vi "ProtocolControl_QMH.vi"() -> ()   [LabVIEW 2015]
uses:
  ProtocolStatus.ctl
  <vilib>/xml/Close Reference(Node).vi
  <vilib>/xml/Load XML File.vi
  <vilib>/xml/NI_XML.lvlib
  <resource>/objmgr/DOMUserDefRef.rc
panel:
  out "Current Subsession":string caption="Name"
  out "Time of Current Subsession":dbl caption="Time"
  out "Current Subsession Idx":i32 caption="Index"
  in  "Engage":bool
  in  "Subject ID":string
  out "Time to Next Subsession":dbl
  out "Pause Time":dbl
  out "Record Time":dbl
  out "Session Time (s)":dbl
  out "Current Session":dbl(slide) min=0.0 max=600.0 scale=0.0..180.0
  out "Current Time":dbl
  out "File Name":string
  out "Suggestions":string
  in  "Close Protocol":bool
  in  "Pause Session":bool
  in  "Start Session":bool
  in  "Load Protocol":bool
  in  "Sessions":i32(listbox)
  out "parse errors":string
  in  "XML File Path":path=path "D:/JinXin/LabVIEW.git/CAlex2-Controller/Remote VIs/Protocol/TrainingProtocol.xml"
  # "Subsession"
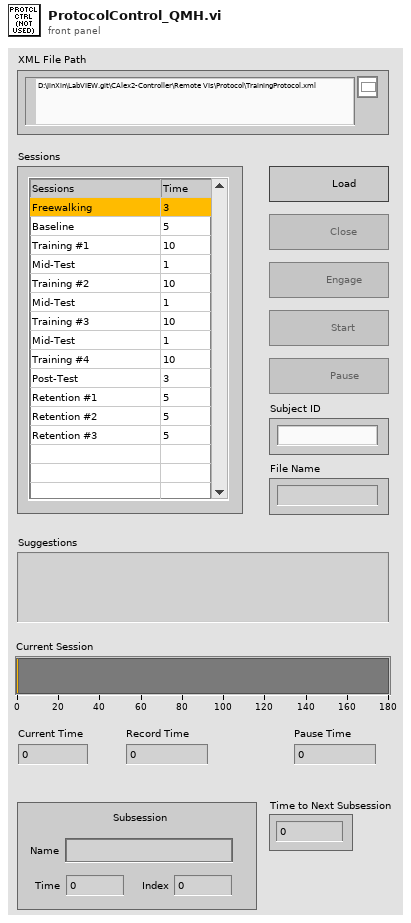
[diagram p1: front panel]
types:
  T1 = typedef "ProtocolStatus.ctl" = enum16{"No Protocol", "Protocol Idle", "Protocol Start", "Protocol Pause"}
  T2 = enum8{"Enabled", "Disabled", "Disabled and Grayed Out"}
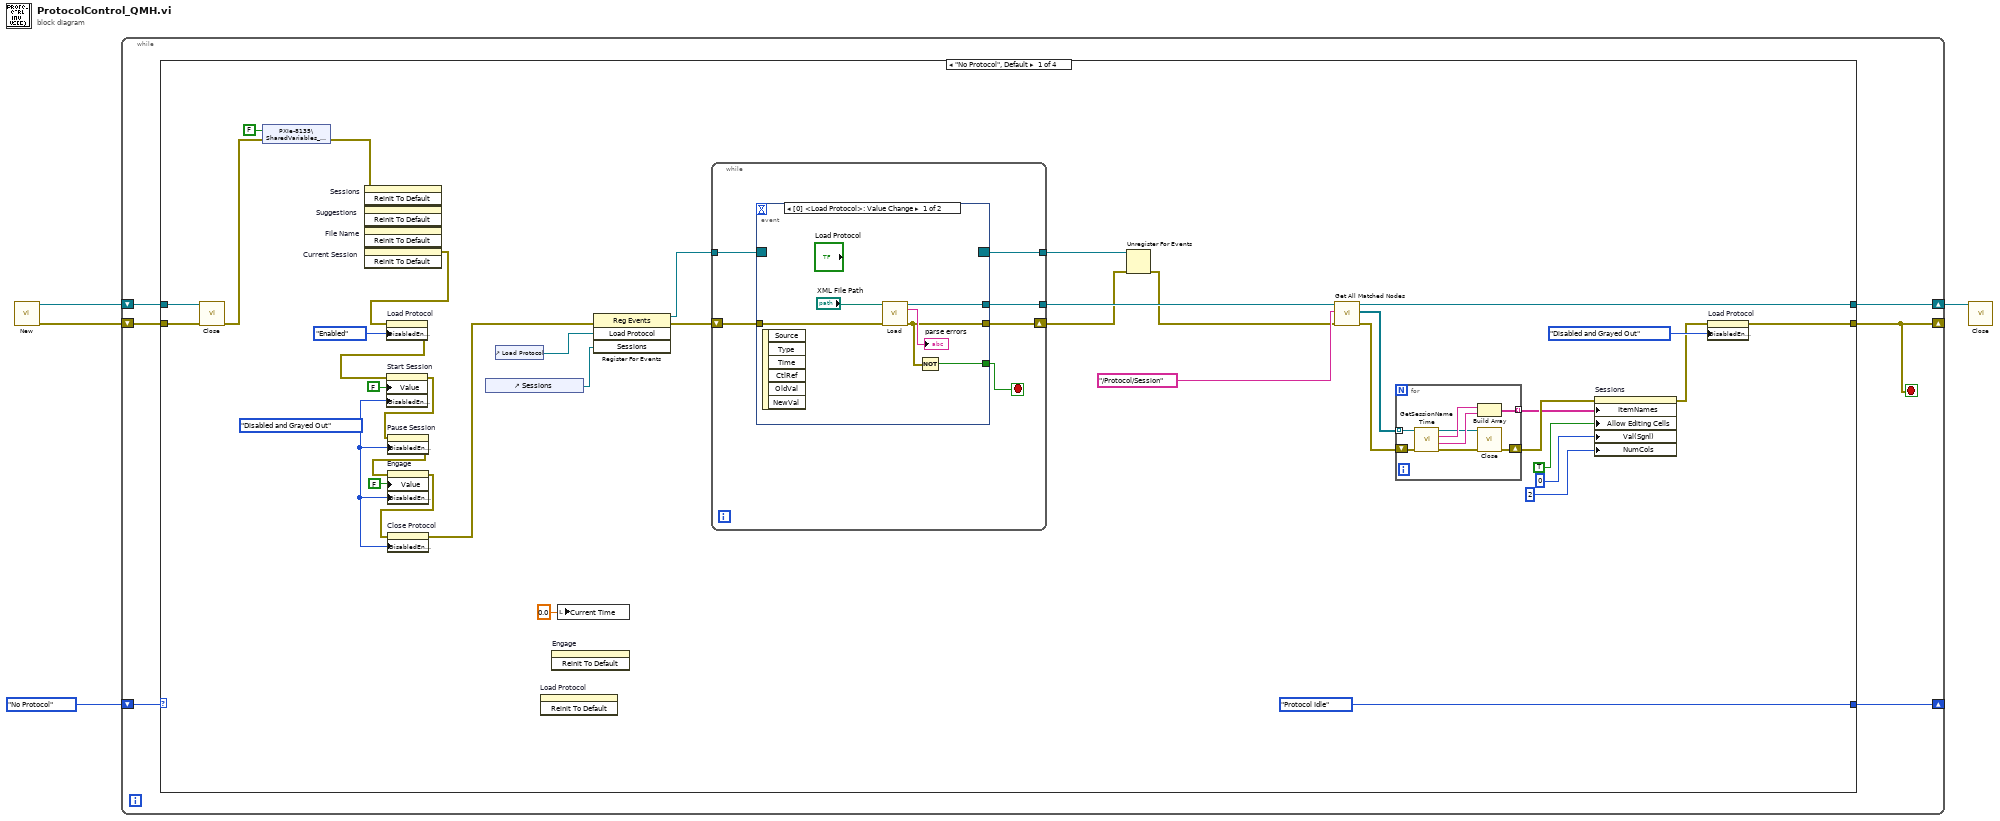
[diagram p0: block diagram]
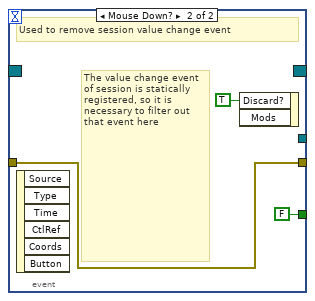
[diagram p2: hidden frame]
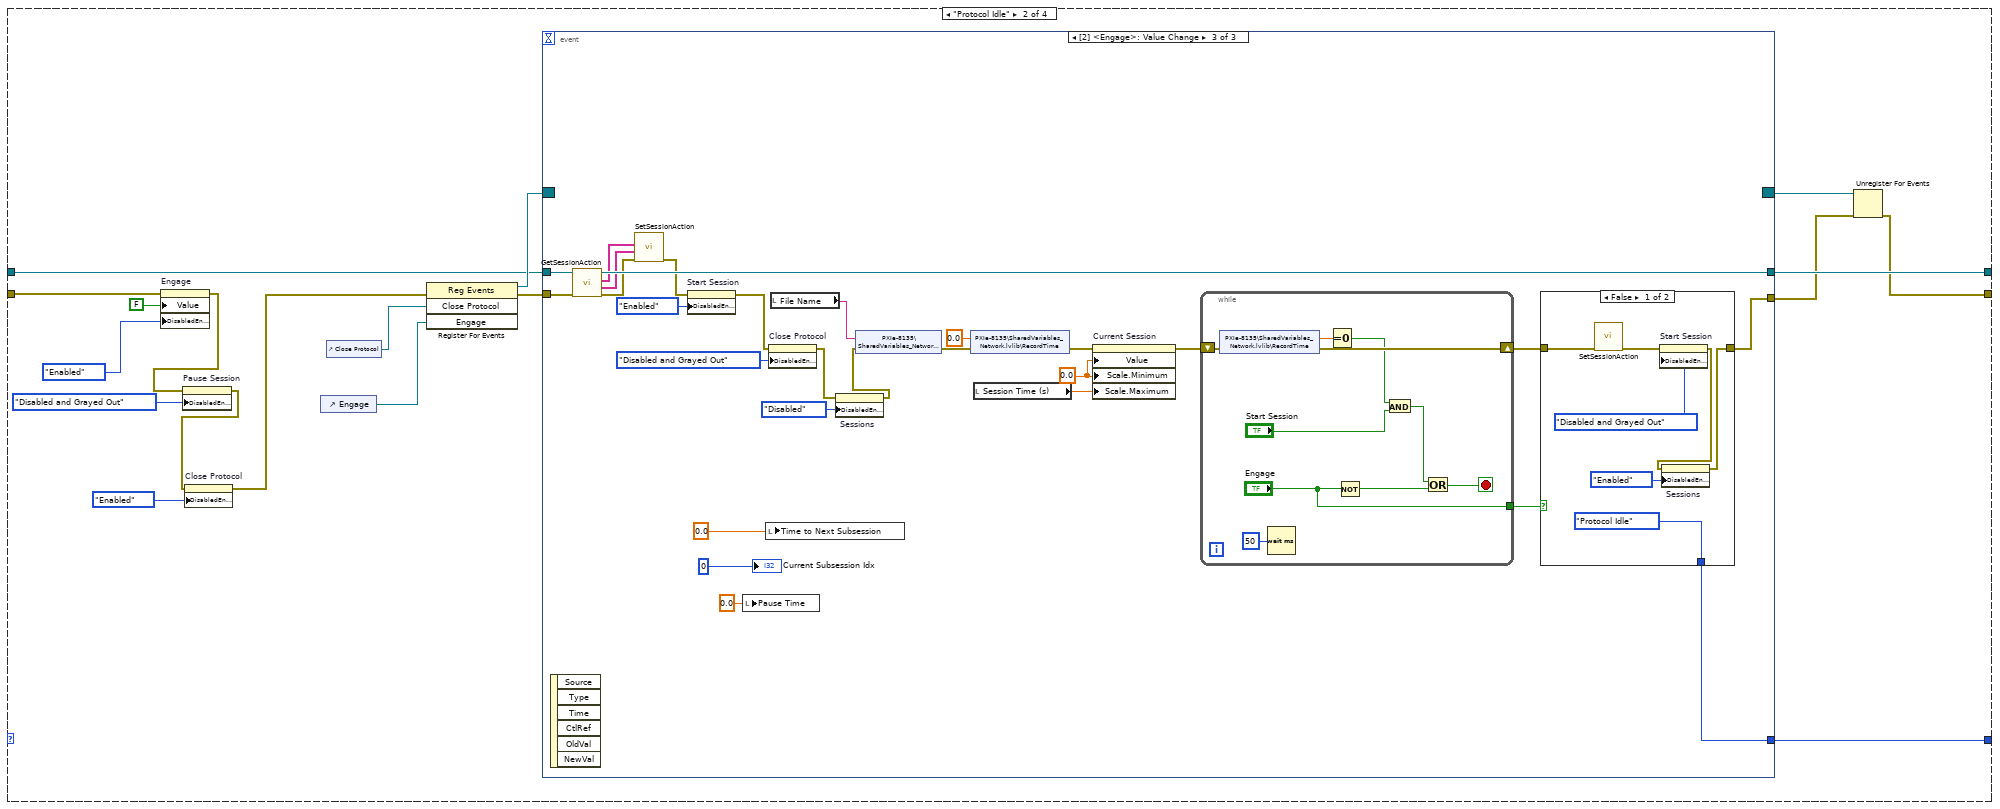
[diagram p3: hidden frame]
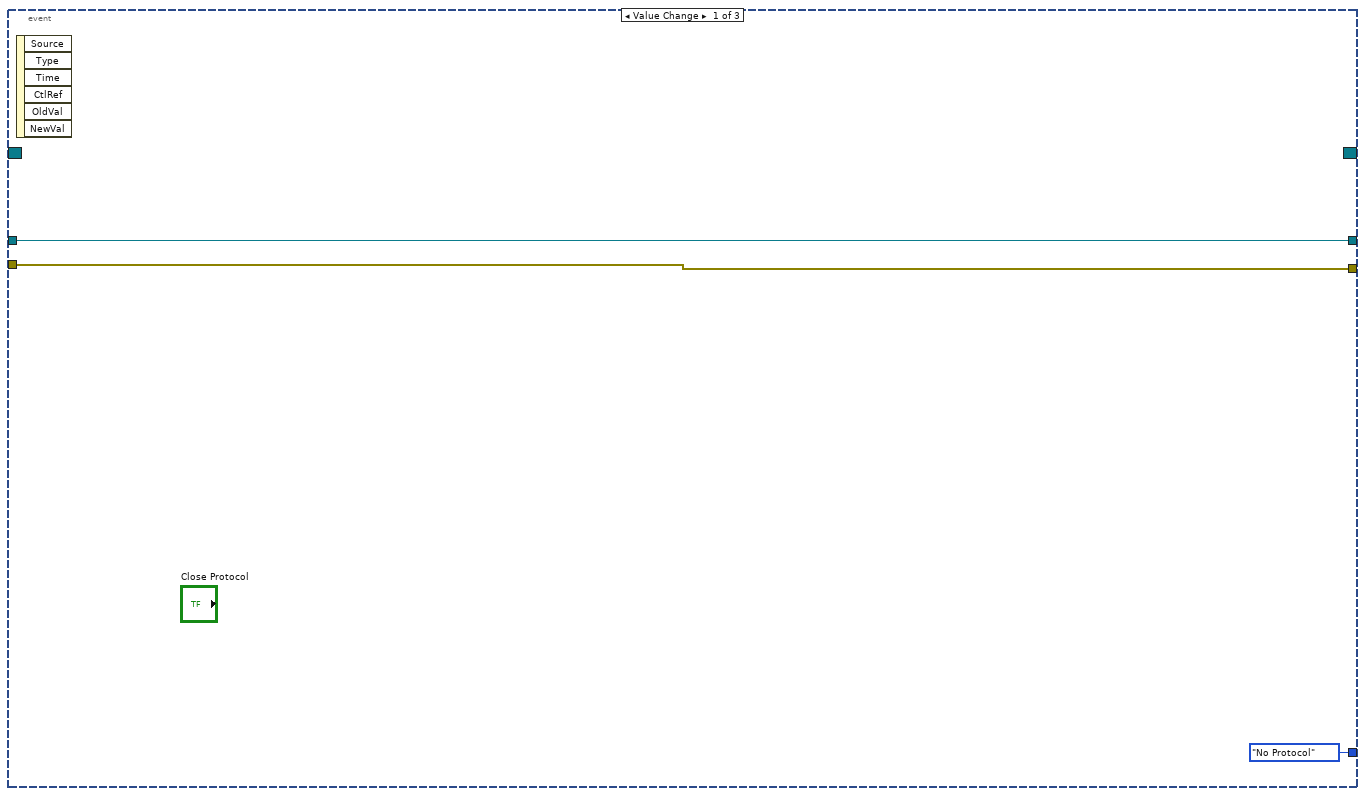
[diagram p4: hidden frame]
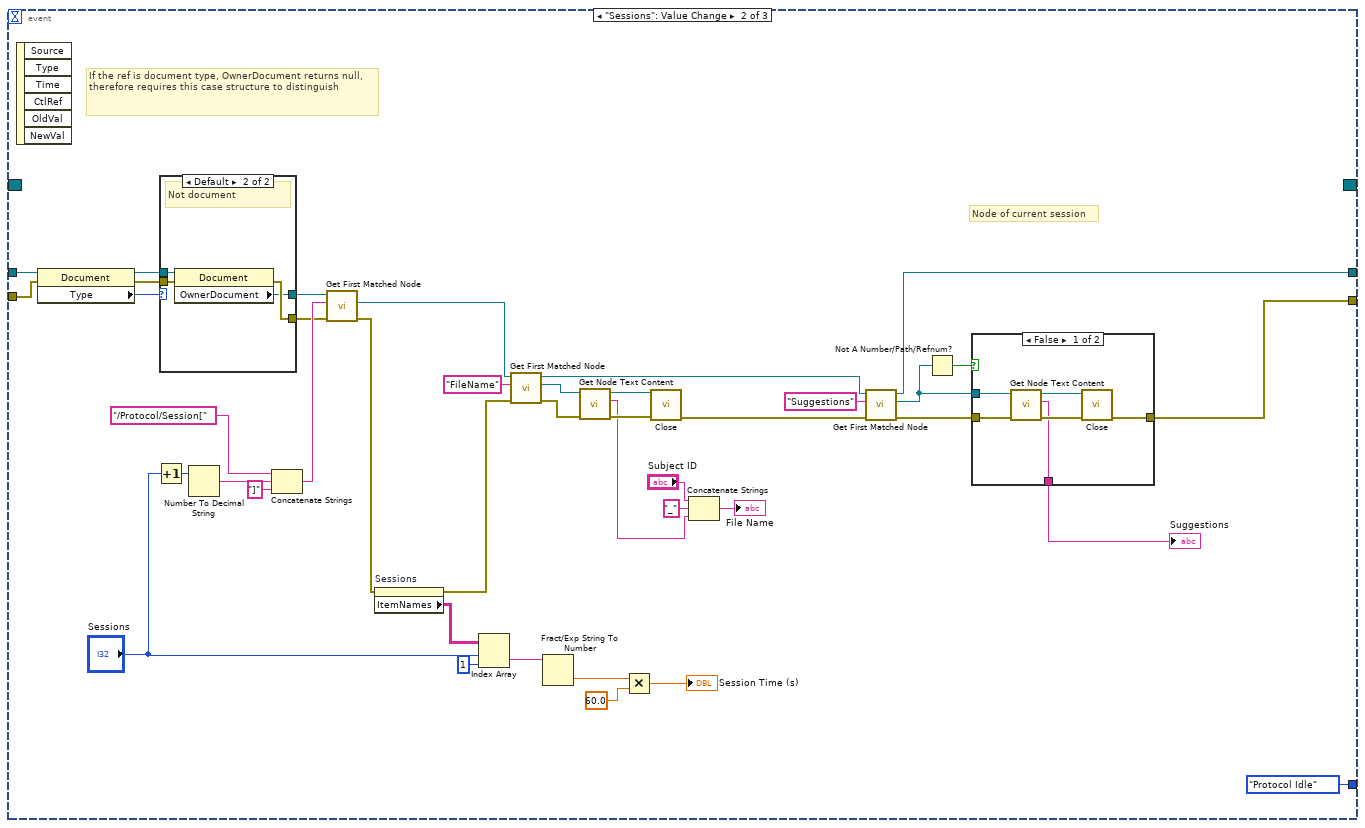
[diagram p5: hidden frame]
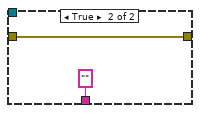
[diagram p7: hidden frame]
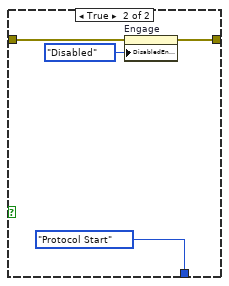
[diagram p8: hidden frame]
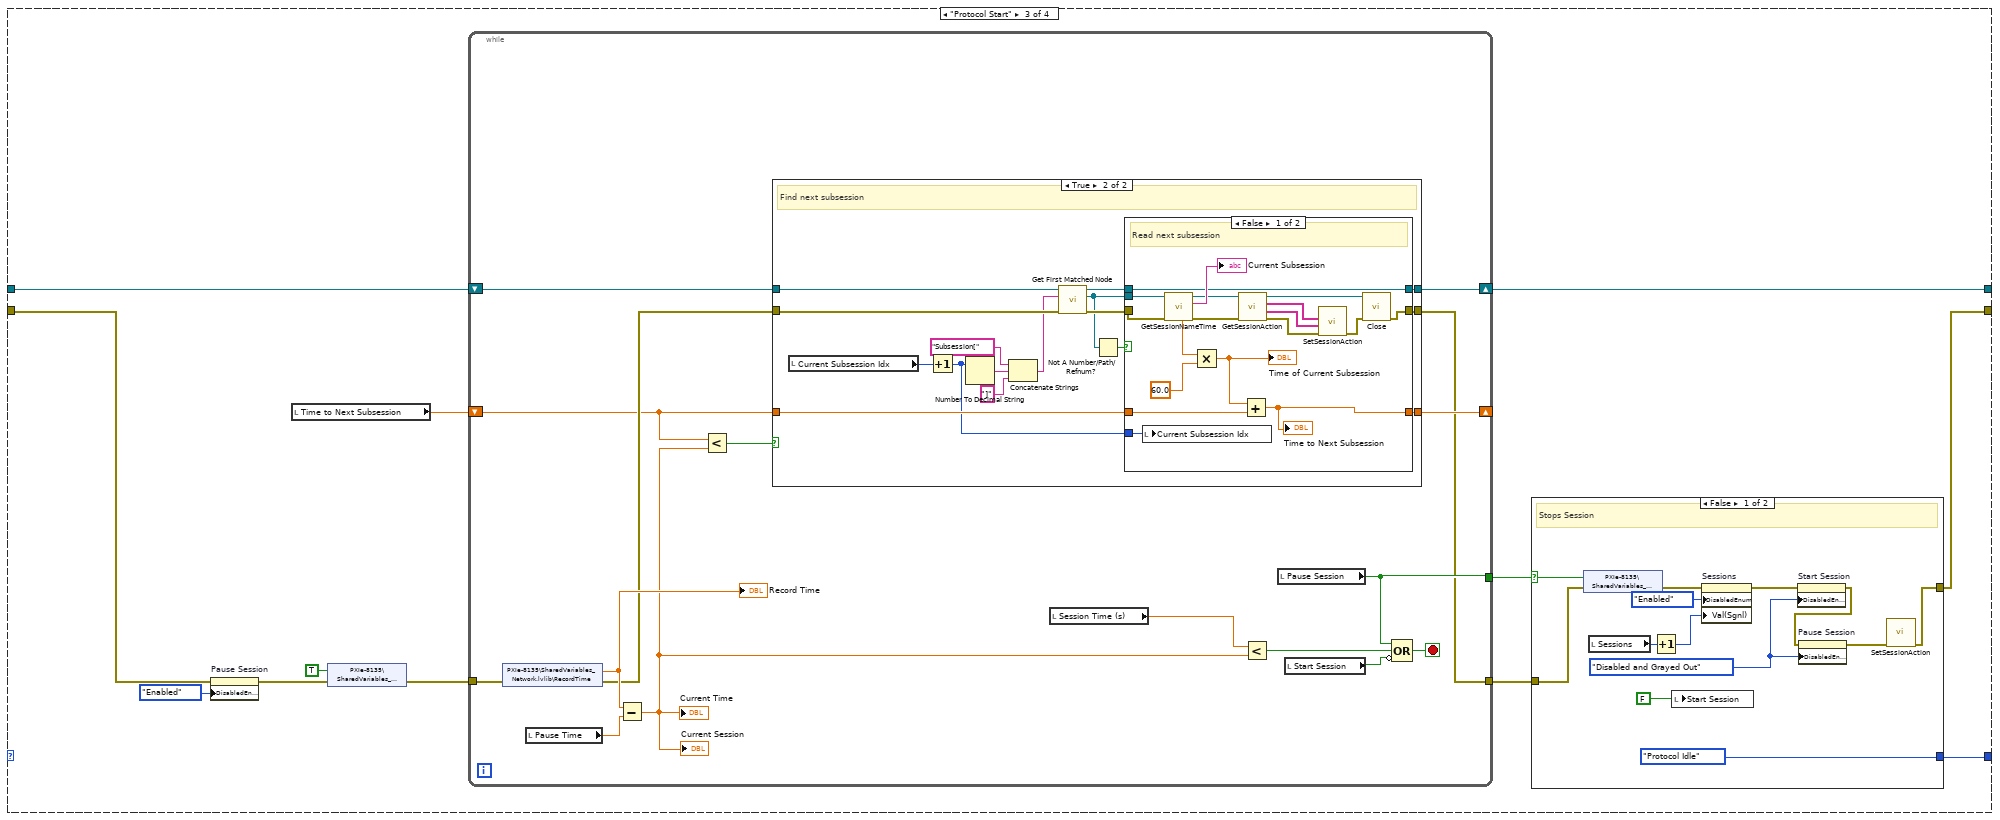
[diagram p9: hidden frame]
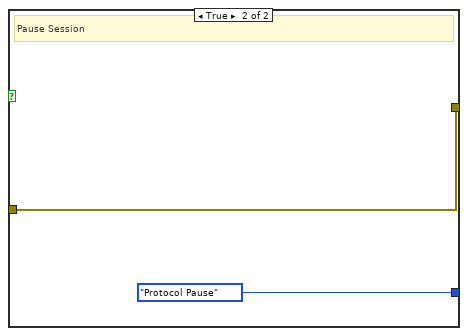
[diagram p10: hidden frame]
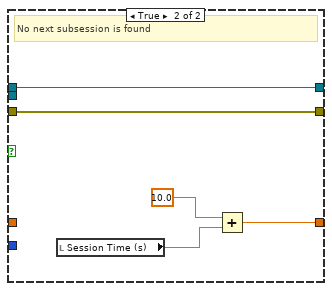
[diagram p12: hidden frame]
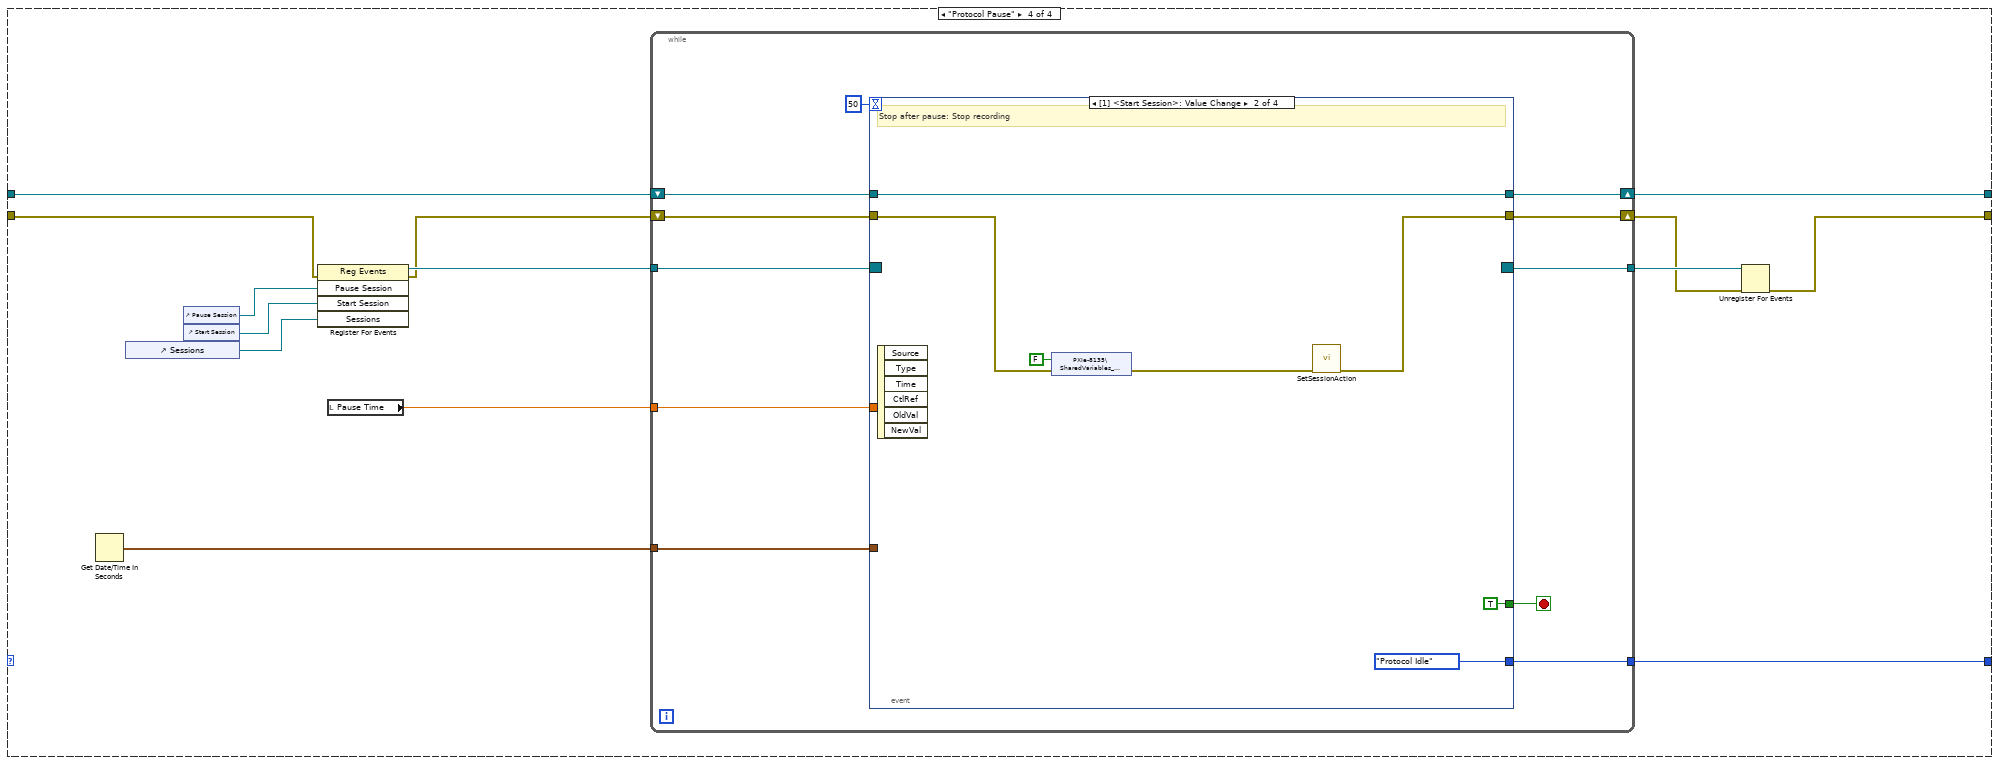
[diagram p13: hidden frame]
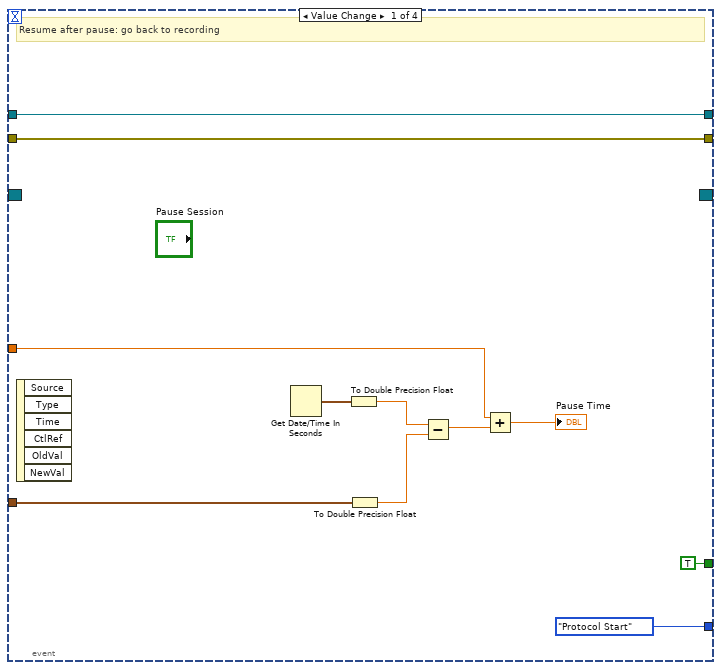
[diagram p14: hidden frame]
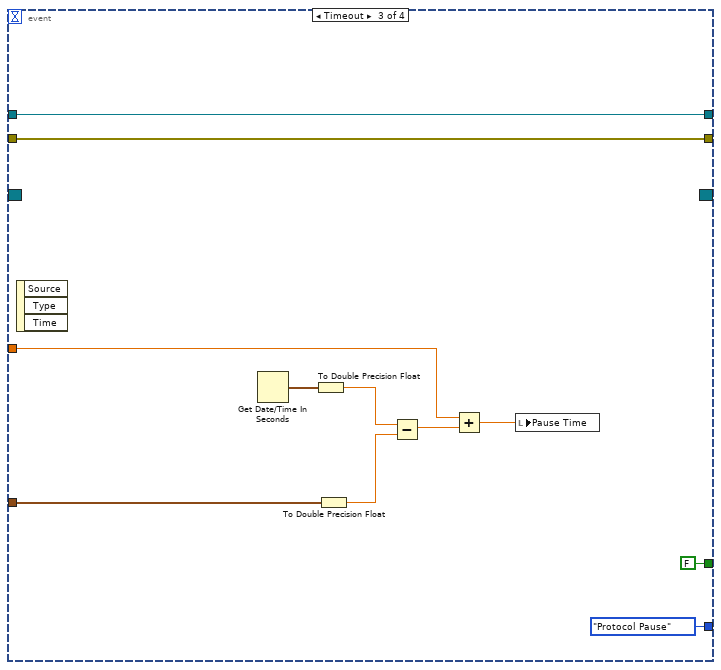
[diagram p15: hidden frame]
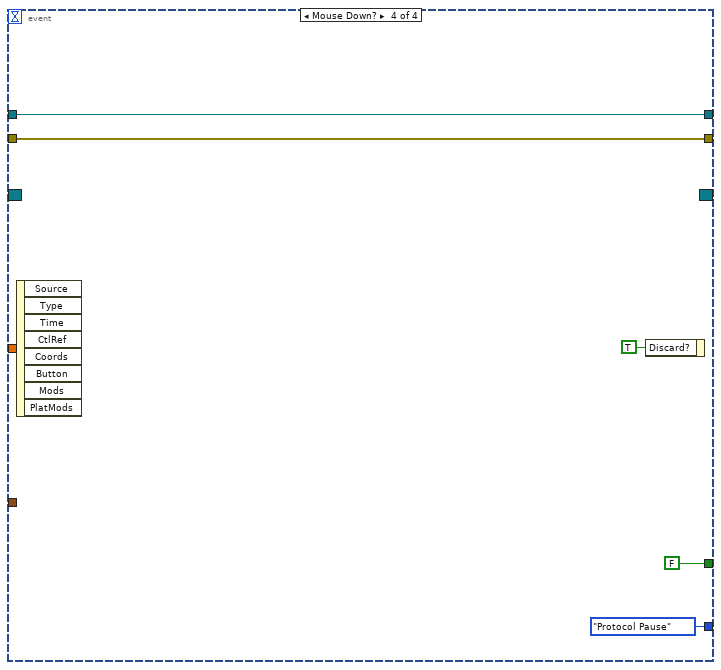
[diagram p16: hidden frame]
diagram:
  n1 = call <vilib>:"New.vi"() -> ("error out"=w2:errorcluster, "DOM document out"=w3:refnum<k20>)  [unwired: 8 in]
  n2 = while {
    shift-right: [w9] -> w1
    shift-left: w3 -> [w8]
    shift-right: [w5] -> _
    shift-left: w2 -> [w7]
    shift-right: [w6] -> _
    shift-left: ProtocolStatus."No Protocol" -> [w10]
    stop <- w5 stop-if-true
    n3 = case shown="\"No Protocol\", Default" w10 {
      tunnel: [w43 w90 w207 w294] -> w9
      tunnel: w8 -> [w50 w85 w200 w295]
      tunnel: w7 -> [w49 w83 w199 w288]
      tunnel: [w13 w75 w204 w284] -> w5
      tunnel: [ProtocolStatus."Protocol Idle" w91 w203 w296] -> w6
      frame "No Protocol", Default {
        w14 = T2."Disabled and Grayed Out" ("Disabled")
        n4 = call-poly <vilib>:"Close.vi"("error in (no error)"=w49, "node"=w50) -> ("error out"=w28:errorcluster)  [unwired: 7 in]
        n5 = shared-variable "PXIe-8135\\SharedVariables_Network.lvlib\\Record?"(FALSE ("Record?"), error in=w28) -> (error out=w27:errorcluster)
        n6 = invoke on="Sessions" class="MCListbox (strict)" method="Reinit To Default"(error in=w27) -> (error out=w37:errorcluster)  [unwired: 2 in, 2 out]
        n7 = invoke on="Suggestions" class="Str" method="Reinit To Default"(error in=w37) -> (error out=w36:errorcluster)  [unwired: 2 in, 2 out]
        n8 = invoke on="File Name" class="Str" method="Reinit To Default"(error in=w36) -> (error out=w35:errorcluster)  [unwired: 2 in, 2 out]
        n9 = invoke on="Current Session" class="Slide (strict)" method="Reinit To Default"(error in=w35) -> (error out=w32:errorcluster)  [unwired: 2 in, 2 out]
        n10 = property on="Load Protocol" class="Bool"(error in=w32, "DisabledEnum"=T2."Enabled" ("Disabled")) -> (error out=w26:errorcluster)  [unwired: 1 in, 1 out]
        n11 = property on="Start Session" class="Bool (strict)"(error in=w26, "Value"=FALSE ("Start Session"), "DisabledEnum"=w14) -> (error out=w18:errorcluster)  [unwired: 1 in, 1 out]
        n12 = property on="Pause Session" class="Bool (strict)"(error in=w18, "DisabledEnum"=w14) -> (error out=w17:errorcluster)  [unwired: 1 in, 1 out]
        n13 = property on="Engage" class="Bool (strict)"(error in=w17, "Value"=FALSE ("Engage"), "DisabledEnum"=w14) -> (error out=w16:errorcluster)  [unwired: 1 in, 1 out]
        n14 = property on="Close Protocol" class="Bool"(error in=w16, "DisabledEnum"=w14) -> (error out=w15:errorcluster)  [unwired: 1 in, 1 out]
        n15 = control-ref of="Sessions"() -> (w25:refnum<vi>)
        n16 = control-ref of="Load Protocol"() -> (w24:refnum<vi>)
        n17 = invoke on="Load Protocol" class="Bool" method="Reinit To Default"() -> ()  [unwired: 3 in, 3 out]
        n18 = invoke on="Engage" class="Bool (strict)" method="Reinit To Default"() -> ()  [unwired: 3 in, 3 out]
        n19 = local write "Current Time"(0.0 ("Current Time")) -> ()
        n20 = register-events(error in=w15, w24, w25) -> (reference out=w22:refnum<event-registration>, error out=w23:errorcluster)  [unwired: 1 in]
        n21 = while {
          tunnel: [w56] -> w44
          shift-right: [w53] -> w20
          shift-left: w23 -> [w51]
          tunnel: w22 -> [w54]
          tunnel: [w52] -> w21
          stop <- w55 stop-if-true
          n22 = event shown="[0] <Load Protocol>: Value Change" {
            selector: w54 -> [_ _]
            dyn-events: [_ _] -> w52
            timeout: _ -> [_ _]
            tunnel: [w60 _] -> w56
            tunnel: w51 -> [w59 w63]
            tunnel: [w58 FALSE] -> w55
            tunnel: [w57 w63] -> w53
            event Value Change {
              n23 = event-data() -> ()  [unwired: 1 in, 6 out]
              n24 = call-poly <vilib>:"Load.vi"("path to XML document"="XML File Path", "error in (no error)"=w59) -> ("DOM document out"=w60:refnum<k20>, "parse errors"=→"parse errors":string, "error out"=w57:errorcluster)  [unwired: 11 in]
              n25 = Not(x=w57) -> (.not. x?=w58:bool)
            }
            event Mouse Down? {
              # "The value change event of session is statically registered, so it is necessary to filter out that event here"
              # "Used to remove session value change event"
              n26 = event-data() -> ()  [unwired: 1 in, 6 out]
              n27 = event-data("Discard?"=TRUE) -> ()  [unwired: 2 in, 1 out]
            }
          }
        }
        n28 = Unregister For Events(event registration refnum=w21, error in=w20) -> (error out=w19:errorcluster)
        n29 = call <vilib>:"Get All Matched Nodes.vi"("error in (no error)"=w19, "XPath expression"="/Protocol/Session", "node in"=w44) -> ("error out"=w47:errorcluster, "node result array"=w45:refnum<k20>[], "node out"=w43:refnum<k20>)  [unwired: 6 in]
        n30 = for {
          tunnel: w45 -> [w66] mode=indexing
          shift-right: [w67] -> w42
          shift-left: w47 -> [w73]
          tunnel: [w70] -> w38 mode=indexing
          n31 = call "GetSessionNameTime.vi"("error in (no error)"=w73, "Refnum in"=w66) -> ("error out"=w69:errorcluster, "Session Time"=w72:string, "Session Name"=w71:string, "node out"=w68:refnum<k20>)  [unwired: 5 in, 1 out]
          n32 = Build Array(w71, w72) -> (w70:string[])
          n33 = call-poly <vilib>:"Close.vi"("error in (no error)"=w69, "node"=w68) -> ("error out"=w67:errorcluster)  [unwired: 7 in]
        }
        n34 = property on="Sessions" class="MCListbox (strict)"(error in=w42, "ItemNames"=w38, "Allow Editing Cells"=TRUE, "Val(Sgnl)"=0 ("Protocol"), "NumCols"=u32 2 ("Number of Columns")) -> (error out=w30:errorcluster)  [unwired: 1 in, 1 out]
        n35 = property on="Load Protocol" class="Bool"(error in=w30, "DisabledEnum"=T2."Disabled and Grayed Out" ("Disabled")) -> (error out=w13:errorcluster)  [unwired: 1 in, 1 out]
      }
      frame "Protocol Idle" {
        n36 = property on="Engage" class="Bool (strict)"(error in=w83, "Value"=FALSE ("Engage"), "DisabledEnum"=T2."Enabled" ("Disabled")) -> (error out=w80:errorcluster)  [unwired: 1 in, 1 out]
        n37 = property on="Pause Session" class="Bool (strict)"(error in=w80, "DisabledEnum"=T2."Disabled and Grayed Out" ("Disabled")) -> (error out=w77:errorcluster)  [unwired: 1 in, 1 out]
        n38 = property on="Close Protocol" class="Bool"(error in=w77, "DisabledEnum"=T2."Enabled" ("Disabled")) -> (error out=w74:errorcluster)  [unwired: 1 in, 1 out]
        n39 = control-ref of="Engage"() -> (w84:refnum<vi>)
        n40 = control-ref of="Close Protocol"() -> (w88:refnum<vi>)
        n41 = register-events(error in=w74, w88, w84) -> (reference out=w87:refnum<event-registration>, error out=w89:errorcluster)  [unwired: 1 in]
        n42 = event shown="[2] <Engage>: Value Change" {
          selector: w87 -> [_ _ _]
          dyn-events: [_ _ _] -> w86
          timeout: _ -> [_ _ _]
          tunnel: [ProtocolStatus."No Protocol" ProtocolStatus."Protocol Idle" w162] -> w91
          tunnel: w85 -> [w94 w108 w159]
          tunnel: w89 -> [w93 w107 w158]
          tunnel: [w93 w110 w164] -> w76
          tunnel: [w94 w109 w157] -> w90
          event Value Change {
            n43 = event-data() -> ()  [unwired: 1 in, 6 out]
          }
          event "Sessions": Value Change {
            # "If the ref is document type, OwnerDocument returns null, therefore requires this case structure to distinguish"
            # "Node of current session"
            n44 = event-data() -> ()  [unwired: 1 in, 6 out]
            n45 = property class="Document"(reference=w108, error in=w107) -> (reference out=w103:refnum<k20>, error out=w105:errorcluster, "Type"=w106:i32)
            n46 = Increment(x="Sessions") -> (x+1=w114:i32)
            n47 = case shown="Default" w106 {
              tunnel: [w137 w139] -> w104
              tunnel: w105 -> [w137 w140]
              tunnel: w103 -> [w136 w141]
              tunnel: [w136 w138] -> w102
              frame 9 {
                # "Document Type"
              }
              frame Default {
                # "Not document"
                n48 = property class="Document"(reference=w141, error in=w140) -> (error out=w139:errorcluster, "OwnerDocument"=w138:refnum<k20>)  [unwired: 1 out]
              }
            }
            n49 = Number To Decimal String(number=w114) -> (decimal integer string=w117:string)  [unwired: 1 in]
            n50 = Concatenate Strings("/Protocol/Session[" ("XPath expression"), w117, "]" ("string")) -> (w116:string)
            n51 = call <vilib>:"Get First Matched Node.vi"("error in (no error)"=w104, "XPath expression"=w116, "node in"=w102) -> ("error out"=w112:errorcluster, "node result"=w111:refnum<k20>)  [unwired: 6 in, 1 out]
            n52 = property on="Sessions" class="MCListbox (strict)"(error in=w112) -> (error out=w118:errorcluster, "ItemNames"=w123:string[][])  [unwired: 1 in, 1 out]
            n53 = Index Array(array=w123, index (row)="Sessions", index (col)=1 ("disabled index (col)")) -> (element=w121:string)
            n54 = call <vilib>:"Get First Matched Node.vi"("error in (no error)"=w118, "XPath expression"="FileName", "node in"=w111) -> ("error out"=w133:errorcluster, "node result"=w134:refnum<k20>, "node out"=w124:refnum<k20>)  [unwired: 6 in]
            n55 = Fract/Exp String To Number(string=w121) -> (number=w120:dbl)  [unwired: 3 in, 1 out]
            n56 = call <vilib>:"Get Node Text Content.vi"("error in (no error)"=w133, "node in"=w134) -> ("error out"=w132:errorcluster, "node text"=w98:string, "node out"=w131:refnum<k20>)  [unwired: 7 in]
            n57 = Multiply(x=w120, y=60.0) -> (x*y=→"Session Time (s)":dbl)
            n58 = call-poly <vilib>:"Close.vi"("error in (no error)"=w132, "node"=w131) -> ("error out"=w119:errorcluster)  [unwired: 7 in]
            n59 = Concatenate Strings("Subject ID", "_" ("string"), w98) -> (→"File Name":string)
            n60 = call <vilib>:"Get First Matched Node.vi"("error in (no error)"=w119, "XPath expression"="Suggestions", "node in"=w124) -> ("error out"=w129:errorcluster, "node result"=w127:refnum<k20>, "node out"=w109:refnum<k20>)  [unwired: 6 in]
            n61 = Not A Number/Path/Refnum?(number/path/refnum=w127) -> (NaN/Path/Refnum?=w126:bool)
            n62 = case shown="False" w126 {
              tunnel: w129 -> [w145 w149]
              tunnel: w127 -> [w144 _]
              tunnel: [w143 "" ("node text")] -> w125
              tunnel: [w142 w149] -> w110
              frame False {
                n63 = call <vilib>:"Get Node Text Content.vi"("error in (no error)"=w145, "node in"=w144) -> ("error out"=w146:errorcluster, "node text"=w143:string, "node out"=w147:refnum<k20>)  [unwired: 7 in]
                n64 = call-poly <vilib>:"Close.vi"("error in (no error)"=w146, "node"=w147) -> ("error out"=w142:errorcluster)  [unwired: 7 in]
              }
              frame True {
              }
            }
            "Suggestions" <- w125
          }
          event Value Change {
            w175 = 0.0 ("Data Entry Limits:Minimum")
            n65 = event-data() -> ()  [unwired: 1 in, 6 out]
            n66 = call "GetSessionAction.vi"("error in (no error)"=w158, "Refnum in"=w159) -> ("error out"=w154:errorcluster, "ActionValue"=w155:string[], "ActionName"=w156:string[], "node out"=w157:refnum<k20>)  [unwired: 6 in]
            n67 = call "SetSessionAction.vi"("error in (no error)"=w154, "ActionValue (False)"=w155, "ActionName  (ForceField)"=w156) -> ("error out"=w153:errorcluster)  [unwired: 8 in]
            n68 = property on="Start Session" class="Bool (strict)"(error in=w153, "DisabledEnum"=T2."Enabled" ("Disabled")) -> (error out=w166:errorcluster)  [unwired: 1 in, 1 out]
            n69 = local write "Pause Time"(0.0 ("Pause Time")) -> ()
            n70 = local write "Time to Next Subsession"(0.0 ("Time to Start Next Subsession")) -> ()
            n71 = property on="Close Protocol" class="Bool"(error in=w166, "DisabledEnum"=T2."Disabled and Grayed Out" ("Disabled")) -> (error out=w152:errorcluster)  [unwired: 1 in, 1 out]
            n72 = local read "File Name"() -> (w170:string)
            n73 = property on="Sessions" class="MCListbox (strict)"(error in=w152, "DisabledEnum"=T2."Disabled" ("Disabled")) -> (error out=w151:errorcluster)  [unwired: 1 in, 1 out]
            n74 = shared-variable "PXIe-8135\\SharedVariables_Network.lvlib\\FileName"(w170, error in=w151) -> (error out=w171:errorcluster)
            n75 = shared-variable "PXIe-8135\\SharedVariables_Network.lvlib\\RecordTime"(0.0 ("RecordTime"), error in=w171) -> (error out=w161:errorcluster)
            n76 = local read "Session Time (s)"() -> (w173:dbl)
            n77 = property on="Current Session" class="Slide (strict)"(error in=w161, "Value"=w175, "Scale.Minimum"=w175, "Scale.Maximum"=w173) -> (error out=w160:errorcluster)  [unwired: 1 in, 1 out]
            n78 = while {
              tunnel: ["Engage"] -> w163
              shift-right: [w196] -> w165
              shift-left: w160 -> [w197]
              stop <- w188 stop-if-true
              n79 = shared-variable "PXIe-8135\\SharedVariables_Network.lvlib\\RecordTime"(error in=w197) -> (w195:dbl, error out=w196:errorcluster)
              n80 = Wait (ms)(milliseconds to wait=u32 50) -> ()  [unwired: 1 out]
              n81 = Equal To 0?(x=w195) -> (x = 0?=w193:bool)
              n82 = Not(x="Engage") -> (.not. x?=w191:bool)
              n83 = And(x=w193, y="Start Session") -> (x .and. y?=w192:bool)
              n84 = Or(x=w192, y=w191) -> (x .or. y?=w188:bool)
            }
            n85 = case shown="False" w163 {
              tunnel: w165 -> [w181 w186]
              tunnel: [w177 w185] -> w164
              tunnel: [ProtocolStatus."Protocol Idle" ProtocolStatus."Protocol Start"] -> w162
              frame False {
                n86 = call "SetSessionAction.vi"("error in (no error)"=w181) -> ("error out"=w180:errorcluster)  [unwired: 10 in]
                n87 = property on="Start Session" class="Bool (strict)"(error in=w180, "DisabledEnum"=T2."Disabled and Grayed Out" ("Disabled")) -> (error out=w178:errorcluster)  [unwired: 1 in, 1 out]
                n88 = property on="Sessions" class="MCListbox (strict)"(error in=w178, "DisabledEnum"=T2."Enabled" ("Disabled")) -> (error out=w177:errorcluster)  [unwired: 1 in, 1 out]
              }
              frame True {
                n89 = property on="Engage" class="Bool (strict)"(error in=w186, "DisabledEnum"=T2."Disabled" ("Disabled")) -> (error out=w185:errorcluster)  [unwired: 1 in, 1 out]
              }
            }
            "Current Subsession Idx" <- 0 ("Current Subsession Idx")
          }
        }
        n90 = Unregister For Events(event registration refnum=w86, error in=w76) -> (error out=w75:errorcluster)
      }
      frame "Protocol Start" {
        n91 = property on="Pause Session" class="Bool (strict)"(error in=w199, "DisabledEnum"=T2."Enabled" ("Disabled")) -> (error out=w202:errorcluster)  [unwired: 1 in, 1 out]
        n92 = local read "Time to Next Subsession"() -> (w198:dbl)
        n93 = shared-variable "PXIe-8135\\SharedVariables_Network.lvlib\\Record?"(TRUE ("Record?"), error in=w202) -> (error out=w209:errorcluster)
        n94 = while {
          tunnel: w209 -> [w240]
          shift-right: [w237] -> _
          shift-left: w198 -> [w225]
          tunnel: [w226] -> w205
          tunnel: [w230] -> w206
          shift-right: [w238] -> w207
          shift-left: w200 -> [w234]
          stop <- w231 stop-if-true
          n95 = shared-variable "PXIe-8135\\SharedVariables_Network.lvlib\\RecordTime"(error in=w240) -> (w236:dbl, error out=w227:errorcluster)
          "Record Time" <- w236
          n96 = local read "Pause Time"() -> (w239:dbl)
          n97 = Subtract(x=w236, y=w239) -> (x-y=w232:dbl)
          "Current Session" <- w232
          "Current Time" <- w232
          n98 = Less?(x=w225, y=w232) -> (x < y?=w233:bool)
          n99 = case shown="True" w233 {
            tunnel: w234 -> [w242 w257]
            tunnel: [w242 w256] -> w238
            tunnel: w225 -> [w243 w259]
            tunnel: [w243 w258] -> w237
            tunnel: w227 -> [w241 w254]
            tunnel: [w241 w253] -> w226
            frame False {
            }
            frame True {
              # "Find next subsession"
              n100 = local read "Current Subsession Idx"() -> (w249:i32)
              n101 = Increment(x=w249) -> (x+1=w244:i32)
              n102 = Number To Decimal String(number=w244) -> (decimal integer string=w248:string)  [unwired: 1 in]
              n103 = Concatenate Strings("Subsession[", w248, "]") -> (w245:string)
              n104 = call <vilib>:"Get First Matched Node.vi"("error in (no error)"=w254, "XPath expression"=w245, "node in"=w257) -> ("error out"=w255:errorcluster, "node result"=w250:refnum<k20>, "node out"=w252:refnum<k20>)  [unwired: 6 in]
              n105 = Not A Number/Path/Refnum?(number/path/refnum=w250) -> (NaN/Path/Refnum?=w251:bool)
              n106 = case shown="False" w251 {
                tunnel: w259 -> [w275 _]
                tunnel: [w260 w281] -> w258
                tunnel: w250 -> [w274 _]
                tunnel: [w270 w278] -> w256
                tunnel: w255 -> [w273 w279]
                tunnel: [w269 w279] -> w253
                tunnel: w252 -> [w270 w278]
                tunnel: w244 -> [w268 _]
                frame False {
                  # "Read next subsession"
                  n107 = local write "Current Subsession Idx"(w268) -> ()
                  n108 = call "GetSessionNameTime.vi"("error in (no error)"=w273, "Refnum in"=w274) -> ("error out"=w263:errorcluster, "Session Name"=→"Current Subsession":string, "node out"=w264:refnum<k20>, "Session Time (min)"=w276:dbl)  [unwired: 5 in, 1 out]
                  n109 = Multiply(x=w276, y=60.0) -> (x*y=w272:dbl)
                  "Time of Current Subsession" <- w272
                  n110 = call "GetSessionAction.vi"("error in (no error)"=w263, "Refnum in"=w264) -> ("error out"=w265:errorcluster, "ActionValue"=w266:string[], "ActionName"=w267:string[], "node out"=w261:refnum<k20>)  [unwired: 6 in]
                  n111 = Add(x=w272, y=w275) -> (x+y=w260:dbl)
                  "Time to Next Subsession" <- w260
                  n112 = call "SetSessionAction.vi"("error in (no error)"=w265, "ActionValue (False)"=w266, "ActionName  (ForceField)"=w267) -> ("error out"=w262:errorcluster)  [unwired: 8 in]
                  n113 = call-poly <vilib>:"Close.vi"("error in (no error)"=w262, "node"=w261) -> ("error out"=w269:errorcluster)  [unwired: 7 in]
                }
                frame True {
                  # "No next subsession is found"
                  n114 = local read "Session Time (s)"() -> (w282:dbl)
                  n115 = Add(x=10.0, y=w282) -> (x+y=w281:dbl)
                }
              }
            }
          }
          n116 = local read "Session Time (s)"() -> (w235:dbl)
          n117 = Less?(x=w235, y=w232) -> (x < y?=w229:bool)
          n118 = local read "Pause Session"() -> (w230:bool)
          n119 = local read "Start Session"() -> (w228:bool)
          n120 = Compound Arithmetic op=OR(w230, w229, invert w228) -> (w231:bool)
        }
        n121 = case shown="False" w206 {
          selector: w206 -> [w222 _]
          tunnel: w205 -> [w221 w223]
          tunnel: [w212 w223] -> w204
          tunnel: [ProtocolStatus."Protocol Idle" ProtocolStatus."Protocol Pause"] -> w203
          frame False {
            w215 = T2."Disabled and Grayed Out" ("Disabled")
            # "Stops Session"
            n122 = shared-variable "PXIe-8135\\SharedVariables_Network.lvlib\\Record?"(w222, error in=w221) -> (error out=w218:errorcluster)
            n123 = local read "Sessions"() -> (w219:i32)
            n124 = Increment(x=w219) -> (x+1=w211:i32)
            n125 = local write "Start Session"(FALSE ("Start Session 2")) -> ()
            n126 = property on="Sessions" class="MCListbox (strict)"(error in=w218, "DisabledEnum"=T2."Enabled" ("Disabled"), "Val(Sgnl)"=w211) -> (error out=w216:errorcluster)  [unwired: 1 in, 1 out]
            n127 = property on="Start Session" class="Bool (strict)"(error in=w216, "DisabledEnum"=w215) -> (error out=w214:errorcluster)  [unwired: 1 in, 1 out]
            n128 = property on="Pause Session" class="Bool (strict)"(error in=w214, "DisabledEnum"=w215) -> (error out=w213:errorcluster)  [unwired: 1 in, 1 out]
            n129 = call "SetSessionAction.vi"("error in (no error)"=w213) -> ("error out"=w212:errorcluster)  [unwired: 10 in]
          }
          frame True {
            # "Pause Session"
          }
        }
      }
      frame "Protocol Pause" {
        n130 = Get Date/Time In Seconds() -> (seconds since 1Jan1904=w293:timestamp)
        n131 = control-ref of="Sessions"() -> (w292:refnum<vi>)
        n132 = control-ref of="Pause Session"() -> (w290:refnum<vi>)
        n133 = control-ref of="Start Session"() -> (w291:refnum<vi>)
        n134 = register-events(error in=w288, w290, w291, w292) -> (reference out=w289:refnum<event-registration>, error out=w287:errorcluster)  [unwired: 1 in]
        n135 = local read "Pause Time"() -> (w283:dbl)
        n136 = while {
          tunnel: [w307] -> w296
          shift-right: [w305] -> w294
          shift-left: w295 -> [w306]
          shift-right: [w298] -> w285
          shift-left: w287 -> [w300]
          tunnel: w293 -> [w302]
          tunnel: w289 -> [w301]
          tunnel: [w299] -> w286
          tunnel: w283 -> [w297]
          stop <- w304 stop-if-true
          n137 = event shown="[1] <Start Session>: Value Change" {
            selector: w301 -> [_ _ _ _]
            dyn-events: [_ _ _ _] -> w299
            timeout: 50 -> [_ _ _ _]
            tunnel: [ProtocolStatus."Protocol Start" ProtocolStatus."Protocol Idle" ProtocolStatus."Protocol Pause" ProtocolStatus."Protocol Pause"] -> w307
            tunnel: w300 -> [w316 w323 w333 w339]
            tunnel: w306 -> [w317 w324 w334 w340]
            tunnel: [w317 w324 w334 w340] -> w305
            tunnel: [w316 w319 w333 w339] -> w298
            tunnel: w302 -> [w314 _ w328 _]
            tunnel: [TRUE ("Discard?") TRUE ("Discard?") FALSE ("Discard?") FALSE ("Discard?")] -> w304
            tunnel: w297 -> [w308 _ w326 _]
            event Value Change {
              # "Resume after pause: go back to recording"
              n138 = event-data() -> ()  [unwired: 1 in, 6 out]
              n139 = Get Date/Time In Seconds() -> (seconds since 1Jan1904=w315:timestamp)
              n140 = To Double Precision Float(number=w315) -> (double precision float=w312:dbl)
              n141 = To Double Precision Float(number=w314) -> (double precision float=w313:dbl)
              n142 = Subtract(x=w312, y=w313) -> (x-y=w311:dbl)
              n143 = Add(x=w308, y=w311) -> (x+y=→"Pause Time":dbl)
            }
            event Value Change {
              # "Stop after pause: Stop recording"
              n144 = event-data() -> ()  [unwired: 1 in, 6 out]
              n145 = shared-variable "PXIe-8135\\SharedVariables_Network.lvlib\\Record?"(FALSE ("Record?"), error in=w323) -> (error out=w320:errorcluster)
              n146 = call "SetSessionAction.vi"("error in (no error)"=w320) -> ("error out"=w319:errorcluster)  [unwired: 10 in]
            }
            event Timeout {
              n147 = event-data() -> ()  [unwired: 1 in, 3 out]
              n148 = Get Date/Time In Seconds() -> (seconds since 1Jan1904=w332:timestamp)
              n149 = To Double Precision Float(number=w332) -> (double precision float=w330:dbl)
              n150 = To Double Precision Float(number=w328) -> (double precision float=w331:dbl)
              n151 = Subtract(x=w330, y=w331) -> (x-y=w329:dbl)
              n152 = Add(x=w326, y=w329) -> (x+y=w327:dbl)
              n153 = local write "Pause Time"(w327) -> ()
            }
            event Mouse Down? {
              n154 = event-data() -> ()  [unwired: 1 in, 8 out]
              n155 = event-data("Discard?"=TRUE) -> ()  [unwired: 1 in, 1 out]
            }
          }
        }
        n156 = Unregister For Events(event registration refnum=w286, error in=w285) -> (error out=w284:errorcluster)
      }
    }
  }
  n157 = call-poly <vilib>:"Close.vi"("node"=w1) -> ()  [unwired: 8 in, 1 out]
